vi "DS360 Send Message.vi"(2 "timeout ms":u32=25000, 3 "address string":string, 4 "write buffer":string, 7 "source":string, 8 "write mode (send EOI:0)":i32(ring) items=["send EOI with last character of string", "append CR to string and send EOI with CR", "append LF to string and send EOI with LF", "append CR LF to string and send EOI with LF", "append CR to string but do not send EOI", "append LF to string but do not send EOI", "append CR LF to string but do not send EOI", "do not send EOI"], 9 "error in":T1) -> (0 "address out":string, 1 "byte count":i32, 5 "status":bool[](array[boolean]), 6 "error out":T1)   [LabVIEW 2025, in "MyDS360.lvlib"]
doc: "Sends a string to a message based VXI instrument. In order to communicate with an instrument, you must first open the instrument by running the Open VXI Instrument or running the initialize VI (initialize VIs call the Open VXI Instrument in their block diagram). Use the instrument ID generated by the Open VXI Instrument to address the specific instrument, then set the write mode and enter the string to send. If a write error occurs, error code 1230 is returned. If you fail to open the instrument, error code 1232 is returned."
uses:
  MyDS360.lvlib
panel:
  in  "[empty array]":bool[](array[boolean])
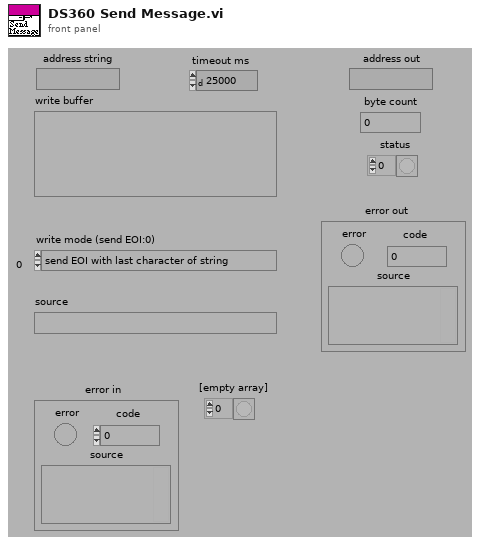
[diagram p1: front panel]
types:
  T1 = cluster{"error":bool, "code":i32, "source":string}
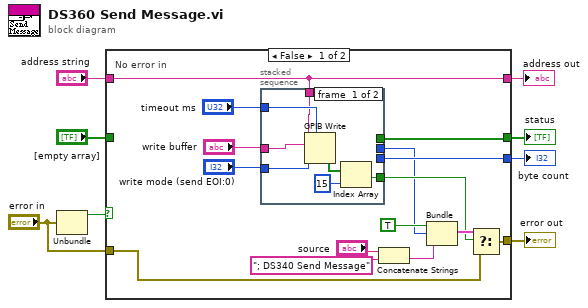
[diagram p0: block diagram]
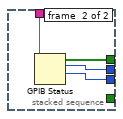
[diagram p2: hidden frame]
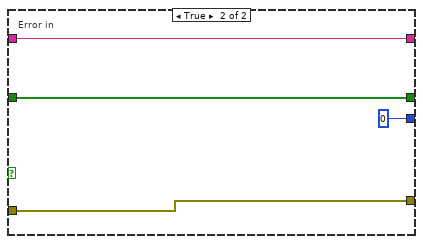
[diagram p3: hidden frame]
diagram:
  n1 = Unbundle("error in") -> ("error"=w6:bool)  [unwired: 2 out]
  n2 = case shown="False" w6 {
    tunnel: "[empty array]" -> [_ w36]
    tunnel: [w16 w36] -> w7
    tunnel: [w22 w37] -> w3
    tunnel: "error in" -> [w13 w37]
    tunnel: [w17 0] -> w8
    tunnel: "address string" -> [w9 w35]
    tunnel: [w9 w35] -> w1
    frame False {
      # "No error in"
      n3 = stacked-sequence {
        tunnel: [_ w33] -> w16
        tunnel: [_ w34] -> w17
        tunnel: [w27 _] -> w18
        tunnel: "write mode (send EOI:0)" -> [w25 _]
        tunnel: "write buffer" -> [w28 _]
        tunnel: [_ w32] -> w15
        tunnel: "timeout ms" -> [w26 _]
        tunnel: w9 -> [w24 w31]
        frame #0 {
          n4 = GPIB Write(0:w24, 1:w28, 2:w25, 4:w26) -> (5:w29:bool[])  [unwired: 1 in, 1 out]
          n5 = Index Array(array=w29, index=15) -> (element=w27:bool)
        }
        frame #1 {
          n6 = GPIB Status(0:w31) -> (2:w33:bool[], 3:w32:i16, 4:w34:i32)  [unwired: 1 in, 1 out]
        }
      }
      n7 = Concatenate Strings("source", "; DS340 Send Message") -> (w14:string)
      n8 = Bundle(TRUE, "GPIB error"=w15, w14) -> (w23:cluster{bool, "GPIB error":i16, string})  [unwired: 1 in]
      n9 = Select(t=w23, s=w18, f=w13) -> (s? t:f=w22:T1)
    }
    frame True {
      # "Error in"
    }
  }
  "status" <- w7
  "byte count" <- w8
  "error out" <- w3
  "address out" <- w1
